vi "Volts To Pressure.vi"(8 "error in (no error)":errorcluster, 9 "Volts":dbl, 10 "Pressure Sensor Settings":T1 {"Offset" format="%_6f"; "PSI per Volt" format="%_6f"}, 11 "Voltage To Pressure in":refnum<class "Voltage To Pressure.lvclass">) -> (0 "error out":errorcluster, 2 "Pressure":dbl, 3 "Voltage To Pressure out":refnum<class "Voltage To Pressure.lvclass">)   [LabVIEW 2015, in "Voltage To Pressure.lvclass"]
uses:
  Voltage To Pressure.lvclass
  Typedefs/Pressure Sensor Settings.ctl
  Typedefs/FAMT Typedefs.lvlib
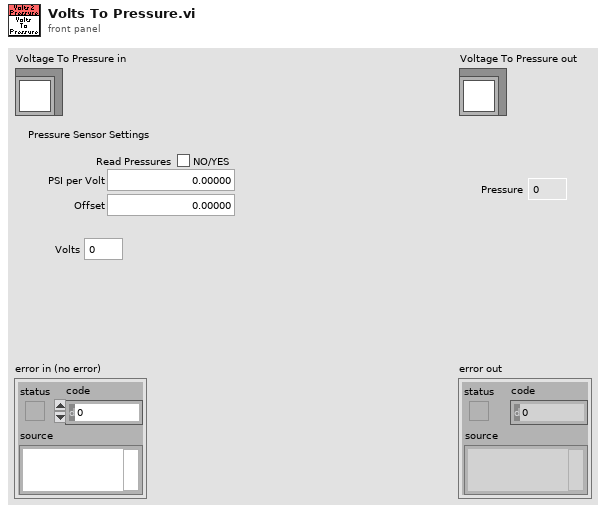
[diagram p1: front panel]
types:
  T1 = typedef "FAMT Typedefs.lvlib/Pressure Sensor Settings.ctl" = cluster{"Read Pressures":bool, "PSI per Volt":dbl, "Offset":dbl}
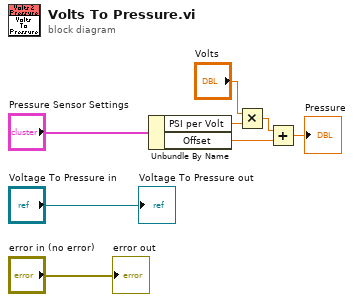
[diagram p0: block diagram]
diagram:
  n1 = Unbundle By Name("Pressure Sensor Settings") -> ("PSI per Volt"=w5:dbl, "Offset"=w6:dbl)
  n2 = Multiply(x="Volts", y=w5) -> (x*y=w7:dbl)
  n3 = Add(x=w7, y=w6) -> (x+y=→"Pressure":dbl)
  "error out" <- "error in (no error)"
  "Voltage To Pressure out" <- "Voltage To Pressure in"
